vi "lift pid.vi"(2 "Setpoint":dbl, 3 "Lift Command":T1) -> (0 "Output":dbl)   [LabVIEW 2014]
uses:
  typedefs/lift/lift command.ctl
  typedefs/safety data/lift safety data.ctl
  global variables/devrefs.vi
  <vilib>/addons/control/pid/pid.llb/PID (DBL).vi
  global variables/safeties.vi
  <vilib>/addons/control/pid/NI_PID_pid.lvlib
panel:
  out "Distance":dbl
  out "Waveform Chart":dbl(graph)
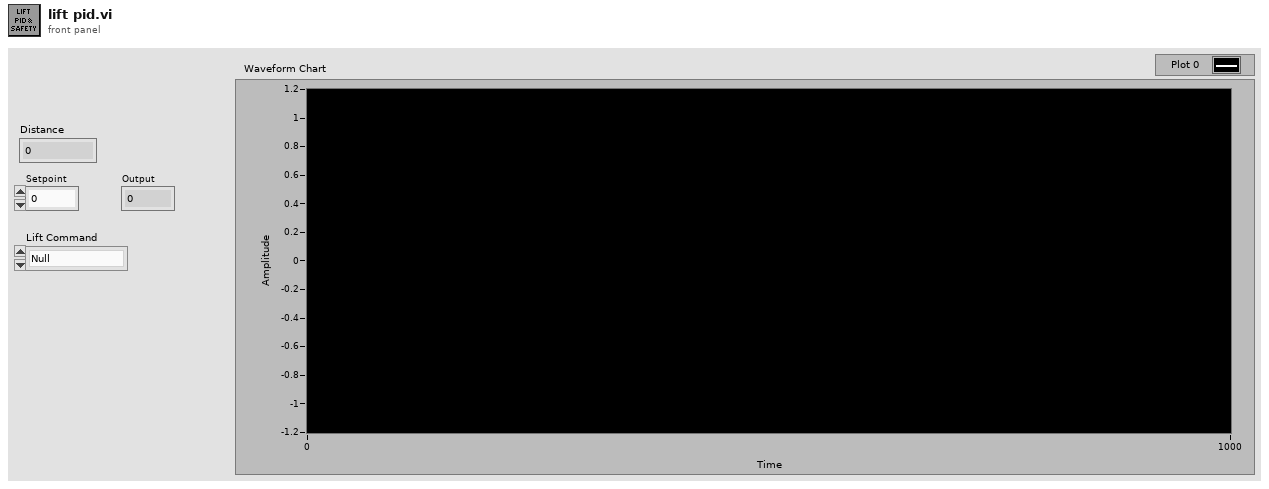
[diagram p1: front panel]
types:
  T1 = typedef "lift command.ctl" = enum16{"Null", "Index Up", "Index Down", "Go To Home", "Pick Up Auto Stack", "Container Index Up", "Container Index Down", "Autonomous"}
  T2 = typedef "lift safety data.ctl" = cluster{"Encoder Disconnected":bool, "At Distance Limit":bool, "Encoder Directional Issue":bool, "Input Out of Range":bool}
  T3 = typedef "WPI_EncoderDevRef.ctl" = cluster{"DevStatus":errorcluster, "EncoderIndex":T4, "CounterIndex":T5, "DistancePerCount":dbl, "Decoding Type":T6}
  T4 = typedef "FPGA_EncoderIdx.ctl" = enum8{"Enc 0", "Enc 1", "Enc 2", "Enc 3", "Enc 4", "Enc 5", "Enc 6", "Enc 7", "Invalid"}
  T5 = typedef "FPGA_CounterCtrSystemIndex.ctl" = enum8{"Ctr 0", "Ctr 1", "Ctr 2", "Ctr 3", "Ctr 4", "Ctr 5", "Ctr 6", "Ctr 7", "Invalid"}
  T6 = typedef "WPI_EncoderType.ctl" = enum16{"1x", "2x", "4x"}
  T7 = typedef "subStates.ctl" = enum16{"null", "wait", "driver control", "auto", "manual override", "hold position", "rotate", "test", "end"}
  T8 = cluster{"proportional gain (Kc)":dbl, "integral time (Ti, min)":dbl, "derivative time (Td, min)":dbl}
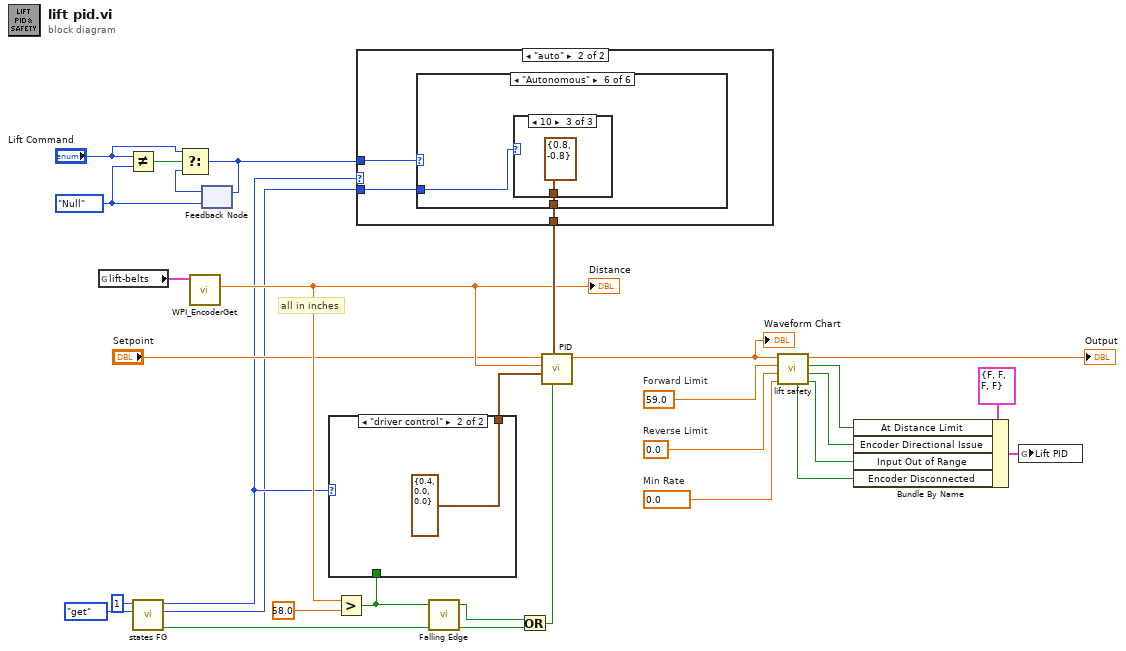
[diagram p0: block diagram]
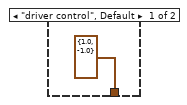
[diagram p2: hidden frame]
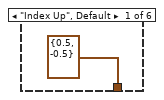
[diagram p3: hidden frame]
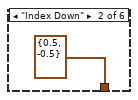
[diagram p4: hidden frame]
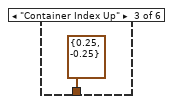
[diagram p5: hidden frame]
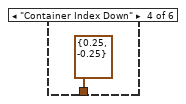
[diagram p6: hidden frame]
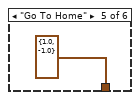
[diagram p7: hidden frame]
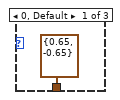
[diagram p8: hidden frame]
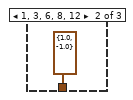
[diagram p9: hidden frame]
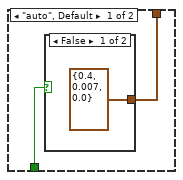
[diagram p10: hidden frame]
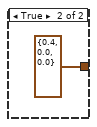
[diagram p11: hidden frame]
diagram:
  w17 = lift_command."Null" ("Lift Command")
  w18 = 0.0  # Min Rate
  w19 = 0.0  # Reverse Limit
  w20 = 59.0  # Forward Limit
  # "all in inches"
  n1 = global read "devrefs.vi" "lift-belts"() -> (w28:T3)
  n2 = Not Equal?(x="Lift Command", y=w17) -> (x != y?=w16:bool)
  n3 = call "states FG.vi"("menu (get)"=enum16{"set", "get"}."get", "Loop ID"=1) -> ("first call?"=w12:bool, "state # out"=w1:i32, "subState out"=w2:T7)  [unwired: 6 in, 1 out]
  n4 = call <vilib>:"WPI_EncoderGet.vi"("EncoderDevRef"=w28) -> ("Distance"=w9:dbl)  [unwired: 5 in, 5 out]
  "Distance" <- w9
  n5 = feedback #1(w17) -> (w15:T1)
  n6 = Select(t="Lift Command", s=w16, f=w15) -> (s? t:f=w13:T1)
  n7 = feedback-in #1(w13) -> ()
  n8 = Greater?(x=w9, y=58.0) -> (0:w3:bool)
  n9 = case shown="\"driver control\"" w2 {
    tunnel: [w31 T8 {"proportional gain (Kc)"=0.4, "integral time (Ti, min)"=0.0, "derivative time (Td, min)"=0.0} ("PID gains")] -> w6
    tunnel: w3 -> [w32 _]
    frame "auto", Default {
      n10 = case shown="False" w32 {
        tunnel: [T8 {"proportional gain (Kc)"=0.4, "integral time (Ti, min)"=0.007, "derivative time (Td, min)"=0.0} ("PID gains") T8 {"proportional gain (Kc)"=0.4, "integral time (Ti, min)"=0.0, "derivative time (Td, min)"=0.0} ("PID gains")] -> w31
        frame False {
        }
        frame True {
        }
      }
    }
    frame "driver control" {
    }
  }
  n11 = case shown="\"auto\"" w2 {
    tunnel: [cluster{"output high":dbl, "output low":dbl} {"output high"=1.0, "output low"=-1.0} ("output range") w39] -> w11
    tunnel: w13 -> [_ w38]
    tunnel: w1 -> [_ w37]
    frame "driver control", Default {
    }
    frame "auto" {
      n12 = case shown="\"Autonomous\"" w38 {
        tunnel: [cluster{"output high":dbl, "output low":dbl} {"output high"=0.5, "output low"=-0.5} ("output range") cluster{"output high":dbl, "output low":dbl} {"output high"=0.5, "output low"=-0.5} ("output range") cluster{"output high":dbl, "output low":dbl} {"output high"=0.25, "output low"=-0.25} ("output range") cluster{"output high":dbl, "output low":dbl} {"output high"=0.25, "output low"=-0.25} ("output range") cluster{"output high":dbl, "output low":dbl} {"output high"=1.0, "output low"=-1.0} ("output range") w46] -> w39
        tunnel: w37 -> [_ _ _ _ _ w45]
        frame "Index Up", Default {
        }
        frame "Index Down" {
        }
        frame "Container Index Up" {
        }
        frame "Container Index Down" {
        }
        frame "Go To Home" {
        }
        frame "Autonomous" {
          n13 = case shown="10" w45 {
            tunnel: [cluster{"output high":dbl, "output low":dbl} {"output high"=0.65, "output low"=-0.65} ("output range") cluster{"output high":dbl, "output low":dbl} {"output high"=1.0, "output low"=-1.0} ("output range") cluster{"output high":dbl, "output low":dbl} {"output high"=0.8, "output low"=-0.8} ("output range")] -> w46
            frame 0, Default {
            }
            frame 1, 3, 6, 8, 12 {
            }
            frame 10 {
            }
          }
        }
      }
    }
  }
  n14 = call "Falling Edge.vi"("Input"=w3) -> ("Output"=w4:bool)  [unwired: 4 in]
  n15 = Or(x=w4, y=w12) -> (x .or. y?=w7:bool)
  n16 = call-poly <vilib>:"PID.vi"("reinitialize? (F)"=w7, "output range"=w11, "PID gains"=w6, "process variable"=w9, "setpoint"="Setpoint") -> ("output"=w10:dbl)  [unwired: 5 in, 1 out]
  "Waveform Chart" <- w10
  n17 = call "lift safety.vi"("Min Rate"=w18, "Reverse Limit"=w19, "Forward Limit"=w20, "Desired Rate"=w10) -> ("Input Out of Range"=w24:bool, "Encoder Directional Issue"=w23:bool, "At Distance Limit"=w22:bool, "Output Rate"=→"Output":dbl, "Encoder Failure"=w25:bool)  [unwired: 3 in]
  n18 = Bundle By Name(cluster=T2 {"Encoder Disconnected"=FALSE, "At Distance Limit"=FALSE, "Encoder Directional Issue"=FALSE, "Input Out of Range"=FALSE} ("Container Arm PID"), "At Distance Limit"=w22, "Encoder Directional Issue"=w23, "Input Out of Range"=w24, "Encoder Disconnected"=w25) -> (w26:T2)
  n19 = global write "safeties.vi" "Lift PID"(w26) -> ()
